vi "PerfFlushCopy.vi"() -> ()   [LabVIEW 2024, in "POTTypedCircularBuffer.Tests.Perf.lvlib"]
uses:
  POTTypedCircularBuffer.Tests.Perf.lvlib
  Type.ctl
  POTTypedCircularBuffer.lvclass/POTTypedCircularBuffer.ctl
  IsFull.vi
  Wrap.vi
  ReadCount.vi
  Reorder.vi
  POTTypedCircularBuffer.lvclass
  <vilib>/Analysis/NI_AALBase.lvlib
panel:
  out "PeakAll mean 2":dbl format="%.2p"
  out "PeakAll mean":dbl format="%.2p"
  out "PeakAll standard deviation":dbl format="%.2p"
  out "PopAll standard deviation":dbl format="%.2p"
  out "PopAll mean":dbl format="%.2p"
  out "Flush standard deviation":dbl format="%.2p"
  out "Flush mean":dbl format="%.2p"
  # "Hard to profile without the compiler being too smart and folding"
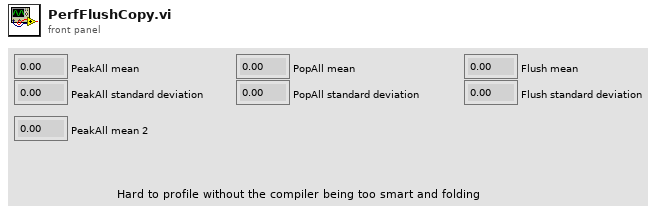
[diagram p1: front panel]
types:
  T1 = typedef "POTTypedCircularBuffer.lvclass/Type.ctl" = i32
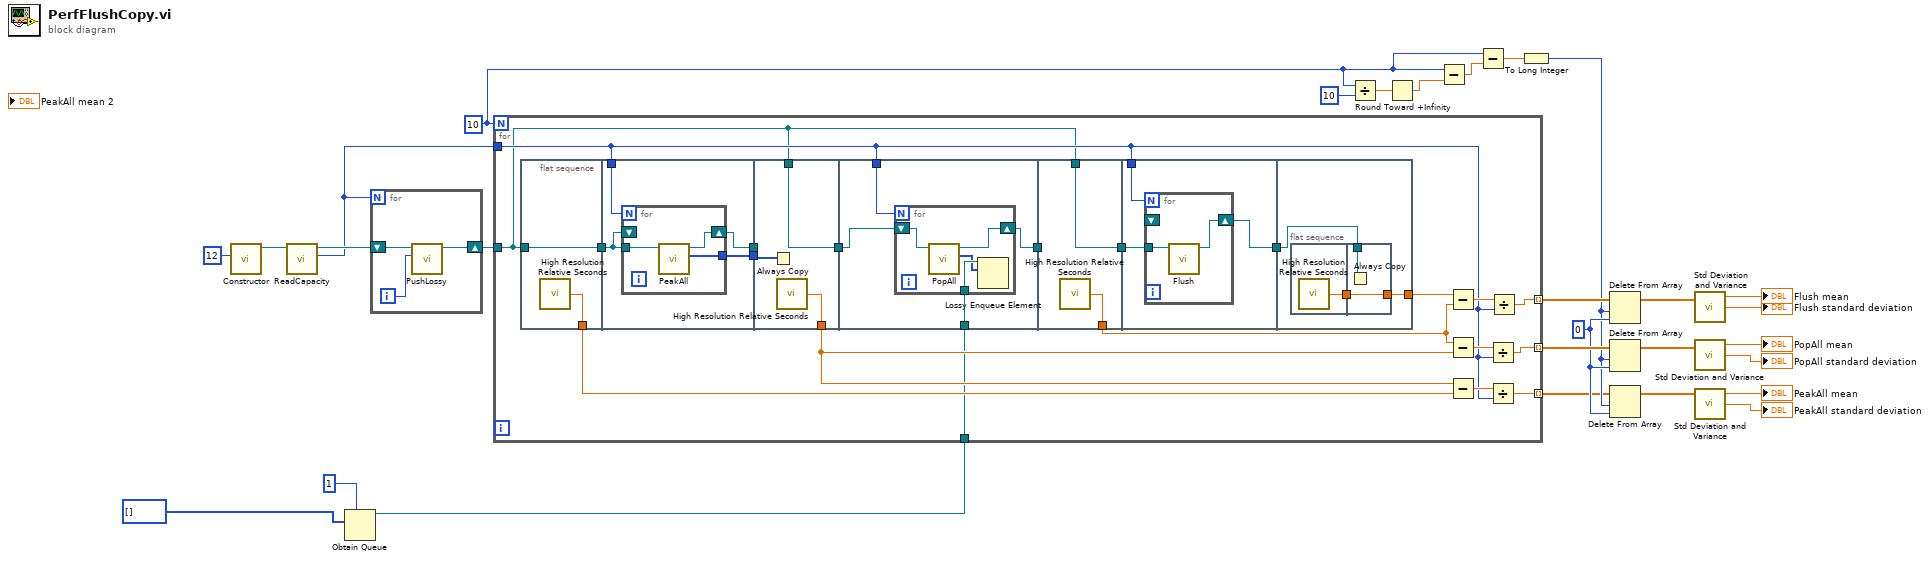
[diagram p0: block diagram]
diagram:
  w12 = 0 ("index")
  w7 = 10
  n1 = call "Constructor.vi"("Capacity 2^n"=u32 12) -> ("POTTypedCircularBuffer out"=w23:refnum<class "POTTypedCircularBuffer.lvclass">)  [unwired: 10 in]
  n2 = call "ReadCapacity.vi"("POTTypedCircularBuffer in"=w23) -> ("capacity"=w21:i32, "POTTypedCircularBuffer out"=w22:refnum<class "POTTypedCircularBuffer.lvclass">)  [unwired: 9 in]
  n3 = Obtain Queue(max queue size (-1, unlimited)=1, element data type=T1[] [] ("Flushed Buffer")) -> (queue out=w2:refnum<queue>)  [unwired: 3 in, 2 out]
  n4 = for {
    N: w21 -> [_]
    shift-right: [w30] -> w20
    shift-left: w22 -> [w31]
    i -> [w29]
    n5 = call "PushLossy.vi"("Element"=w29, "POTTypedCircularBuffer in"=w31) -> ("POTTypedCircularBuffer out"=w30:refnum<class "POTTypedCircularBuffer.lvclass">)  [unwired: 7 in, 2 out]
  }
  n6 = for {
    N: w7 -> [_]
    tunnel: [w45] -> w17 mode=indexing
    tunnel: w20 -> [w34]
    tunnel: [w46] -> w15 mode=indexing
    tunnel: w21 -> [w38]
    tunnel: [w37] -> w4 mode=indexing
    tunnel: w2 -> [w32]
    n7 = flat-sequence {
      tunnel: w34 -> [w53]
      tunnel: [w53] -> w43
      tunnel: [w52] -> w39
      tunnel: w43 -> [w55]
      tunnel: [w54] -> w42
      tunnel: w38 -> [w57]
      tunnel: [w56] -> w36
      tunnel: w42 -> [_]
      tunnel: [w63] -> w40
      tunnel: w36 -> [w62]
      tunnel: w34 -> [w61]
      tunnel: [w61] -> w33
      tunnel: [w67] -> w50
      tunnel: w38 -> [w66]
      tunnel: w33 -> [w65]
      tunnel: w32 -> [w64]
      tunnel: [w73] -> w49
      tunnel: w50 -> [_]
      tunnel: w34 -> [w72]
      tunnel: [w72] -> w35
      tunnel: w38 -> [w76]
      tunnel: [w75] -> w44
      tunnel: w35 -> [w74]
      tunnel: [w81] -> w51
      tunnel: w44 -> [w79]
      frame #0 {
        n8 = call <vilib>:"High Resolution Relative Seconds.vi"() -> ("relative seconds"=w52:dbl)
      }
      frame #1 {
        n9 = for {
          N: w57 -> [_]
          tunnel: [w59] -> w56
          tunnel: w55 -> [w60]
          shift-right: [w58] -> w54
          shift-left: w55 -> [_]
          n10 = call "PeakAll.vi"("POTTypedCircularBuffer in"=w60) -> ("Copied Buffer"=w59:T1[], "POTTypedCircularBuffer out"=w58:refnum<class "POTTypedCircularBuffer.lvclass">)  [unwired: 9 in]
        }
      }
      frame #2 {
        n11 = Always Copy(1:w62) -> ()  [unwired: 1 out]
        n12 = call <vilib>:"High Resolution Relative Seconds.vi"() -> ("relative seconds"=w63:dbl)
      }
      frame #3 {
        n13 = for {
          N: w66 -> [_]
          shift-right: [w71] -> w67
          shift-left: w65 -> [w70]
          tunnel: w64 -> [w69]
          n14 = call "PopAll.vi"("POTTypedCircularBuffer in"=w70) -> ("Flushed Buffer"=w68:T1[], "POTTypedCircularBuffer out"=w71:refnum<class "POTTypedCircularBuffer.lvclass">)  [unwired: 9 in]
          n15 = Lossy Enqueue Element(queue=w69, element=w68) -> ()  [unwired: 1 in, 4 out]
        }
      }
      frame #4 {
        n16 = call <vilib>:"High Resolution Relative Seconds.vi"() -> ("relative seconds"=w73:dbl)
      }
      frame #5 {
        n17 = for {
          N: w76 -> [_]
          shift-right: [w78] -> w75
          shift-left: _ -> [_]
          tunnel: w74 -> [w77]
          n18 = call "Flush.vi"("POTTypedCircularBuffer in"=w77) -> ("POTTypedCircularBuffer out"=w78:refnum<class "POTTypedCircularBuffer.lvclass">)  [unwired: 10 in]
        }
      }
      frame #6 {
        n19 = flat-sequence {
          tunnel: [w82] -> w80
          tunnel: [w84] -> w81
          tunnel: w80 -> [w84]
          tunnel: w79 -> [w83]
          frame #0 {
            n20 = call <vilib>:"High Resolution Relative Seconds.vi"() -> ("relative seconds"=w82:dbl)
          }
          frame #1 {
            n21 = Always Copy(1:w83) -> ()  [unwired: 1 out]
          }
        }
      }
    }
    n22 = Subtract(x=w51, y=w49) -> (x-y=w48:dbl)
    n23 = Subtract(x=w49, y=w40) -> (x-y=w47:dbl)
    n24 = Subtract(x=w40, y=w39) -> (x-y=w41:dbl)
    n25 = Divide(x=w47, y=w38) -> (x/y=w46:dbl)
    n26 = Divide(x=w41, y=w38) -> (x/y=w37:dbl)
    n27 = Divide(x=w48, y=w38) -> (x/y=w45:dbl)
  }
  n28 = Divide(x=w7, y=10) -> (x/y=w10:dbl)
  n29 = Round Toward +Infinity(x=w10) -> (ceil(x): smallest int >= x=w9:dbl)
  n30 = Subtract(x=w7, y=w9) -> (x-y=w6:dbl)
  n31 = Subtract(x=w7, y=w6) -> (x-y=w5:dbl)
  n32 = To Long Integer(number=w5) -> (32bit integer=w8:i32)
  n33 = Delete From Array(array=w17, length=w8, index=w12) -> (array with subset deleted=w16:dbl[])  [unwired: 1 out]
  n34 = Delete From Array(array=w15, length=w8, index=w12) -> (array with subset deleted=w14:dbl[])  [unwired: 1 out]
  n35 = Delete From Array(array=w4, length=w8, index=w12) -> (array with subset deleted=w13:dbl[])  [unwired: 1 out]
  n36 = call <vilib>:"Std Deviation and Variance.vi"("X"=w16) -> ("mean"=→"Flush mean":dbl, "standard deviation"=→"Flush standard deviation":dbl)  [unwired: 1 in, 1 out]
  n37 = call <vilib>:"Std Deviation and Variance.vi"("X"=w14) -> ("mean"=→"PopAll mean":dbl, "standard deviation"=→"PopAll standard deviation":dbl)  [unwired: 1 in, 1 out]
  n38 = call <vilib>:"Std Deviation and Variance.vi"("X"=w13) -> ("mean"=→"PeakAll mean":dbl, "standard deviation"=→"PeakAll standard deviation":dbl)  [unwired: 1 in, 1 out]
